vi "WristDashReadTuningNetwork.vi"() -> (0 "Tune_Kd":dbl, 1 "Tune_Kp":dbl, 2 "Tune_OutMax":dbl, 3 "Tune_OutDb":dbl, 4 "Tune_Kg":dbl, 5 "Tune_ErrDb":dbl, 6 "FilterDerivative":bool, 7 "Tune_ErrThres":dbl, 8 "UseLQR":bool)   [LabVIEW 2023]
uses:
  <vilib>/Rock Robotics/Network Tables/NT Read Number.vi
  <vilib>/Rock Robotics/Network Tables/NT Read Boolean.vi
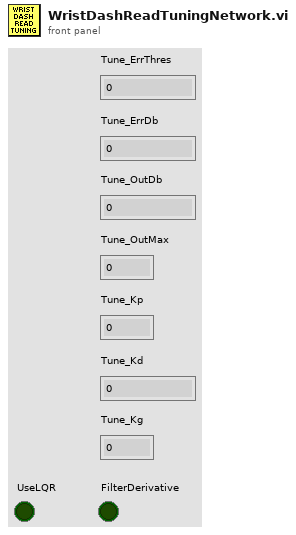
[diagram p1: front panel]
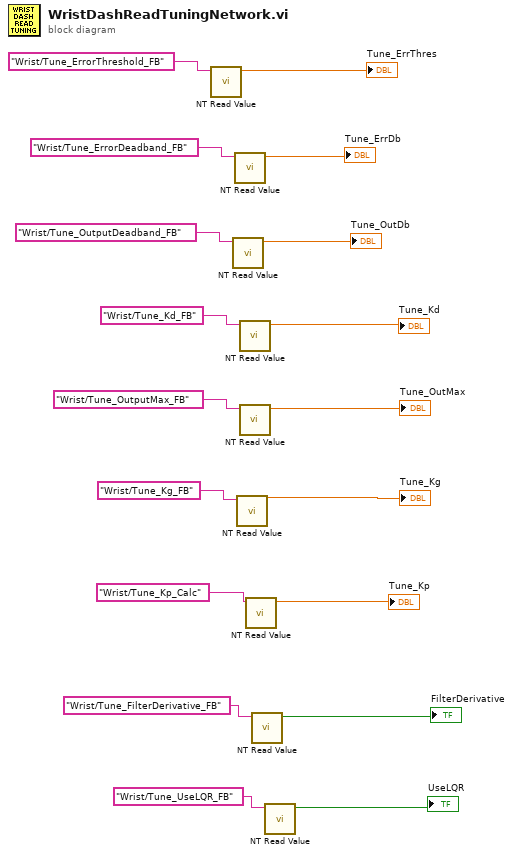
[diagram p0: block diagram]
diagram:
  n1 = call-poly <vilib>:"NT Read Value.vi"("name"="Wrist/Tune_ErrorThreshold_FB") -> ("value"=→"Tune_ErrThres":dbl)  [unwired: 8 in, 2 out]
  n2 = call-poly <vilib>:"NT Read Value.vi"("name"="Wrist/Tune_OutputDeadband_FB") -> ("value"=→"Tune_OutDb":dbl)  [unwired: 8 in, 2 out]
  n3 = call-poly <vilib>:"NT Read Value.vi"("name"="Wrist/Tune_ErrorDeadband_FB") -> ("value"=→"Tune_ErrDb":dbl)  [unwired: 8 in, 2 out]
  n4 = call-poly <vilib>:"NT Read Value.vi"("name"="Wrist/Tune_Kg_FB") -> ("value"=→"Tune_Kg":dbl)  [unwired: 8 in, 2 out]
  n5 = call-poly <vilib>:"NT Read Value.vi"("name"="Wrist/Tune_Kd_FB") -> ("value"=→"Tune_Kd":dbl)  [unwired: 8 in, 2 out]
  n6 = call-poly <vilib>:"NT Read Value.vi"("name"="Wrist/Tune_OutputMax_FB") -> ("value"=→"Tune_OutMax":dbl)  [unwired: 8 in, 2 out]
  n7 = call-poly <vilib>:"NT Read Value.vi"("name"="Wrist/Tune_Kp_Calc") -> ("value"=→"Tune_Kp":dbl)  [unwired: 8 in, 2 out]
  n8 = call-poly <vilib>:"NT Read Value.vi"("name"="Wrist/Tune_FilterDerivative_FB") -> ("value"=→"FilterDerivative":bool)  [unwired: 8 in, 2 out]
  n9 = call-poly <vilib>:"NT Read Value.vi"("name"="Wrist/Tune_UseLQR_FB") -> ("value"=→"UseLQR":bool)  [unwired: 8 in, 2 out]
